vi "Set Preferred Steering Angle.vi"(8 "error in (no error)":errorcluster, 10 "preferred steering angle (rad)":dbl, 11 "wheel in":refnum<class "NI_Robotics_Steering Wheel.lvclass">) -> (0 "error out":errorcluster, 3 "wheel out":refnum<class "NI_Robotics_Steering Wheel.lvclass">)   [LabVIEW 2017, in "NI_Robotics_Steering Wheel.lvclass"]
uses:
  <vilib>/robotics/Steering/Steering Wheel/NI_Robotics_Steering Wheel.lvclass
  <vilib>/robotics/Steering/Steering Wheel/NI_Robotics_Steering Wheel.lvclass/NI_Robotics_Steering Wheel.ctl
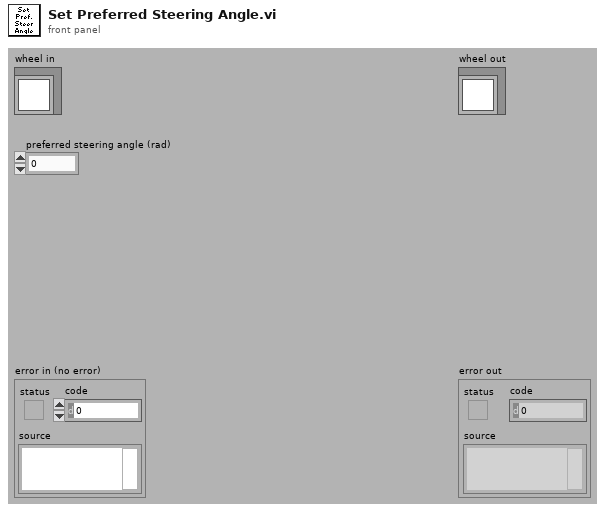
[diagram p1: front panel]
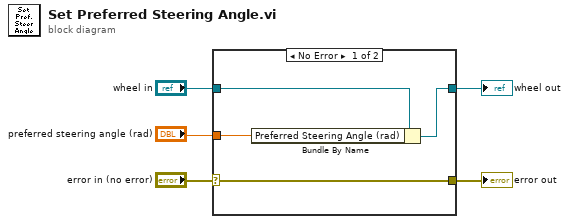
[diagram p0: block diagram]
diagram:
  n1 = case shown="No Error" "error in (no error)" {
    selector: "error in (no error)" -> [w6 w10]
    tunnel: "wheel in" -> [w9 w11]
    tunnel: "preferred steering angle (rad)" -> [w8 _]
    tunnel: [w7 w11] -> w2
    tunnel: [w6 w10] -> w1
    frame No Error {
      n2 = Bundle By Name(cluster=w9, "Preferred Steering Angle (rad)"=w8) -> (w7:refnum<class "NI_Robotics_Steering Wheel.lvclass">)
    }
    frame Error {
    }
  }
  "error out" <- w1
  "wheel out" <- w2
